vi "Trav_Prog_Extra_Commands.vi"() -> (1 "Extra Commands Array":string[](array[string]), 2 "Argument Examples":string[](array[string]))   [LabVIEW 2012]
uses:
  Globals/Extra_Commands_Global.vi
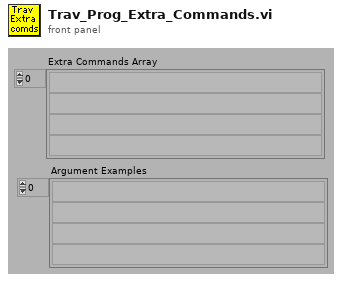
[diagram p1: front panel]
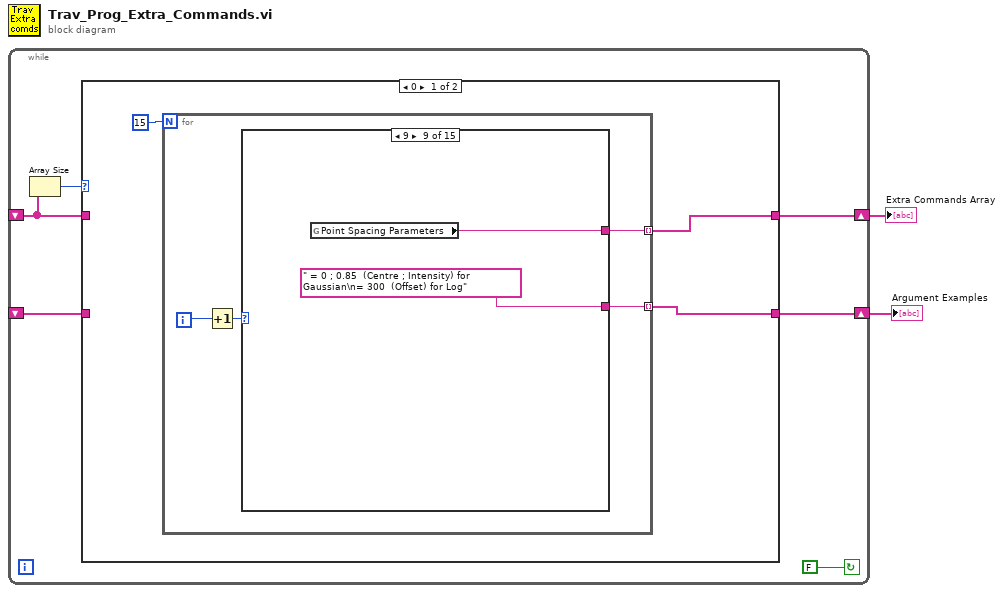
[diagram p0: block diagram]
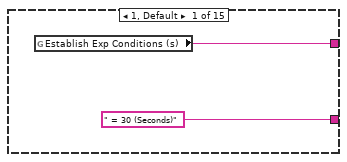
[diagram p2: hidden frame]
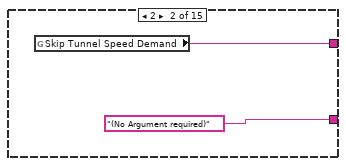
[diagram p3: hidden frame]
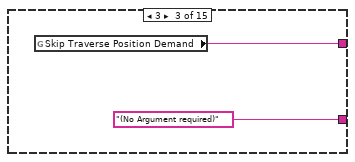
[diagram p4: hidden frame]
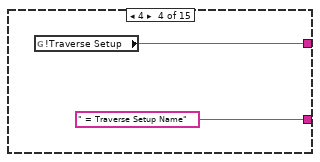
[diagram p5: hidden frame]
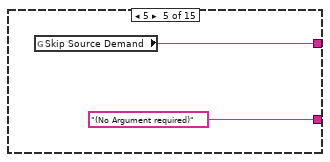
[diagram p6: hidden frame]
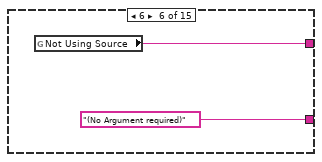
[diagram p7: hidden frame]
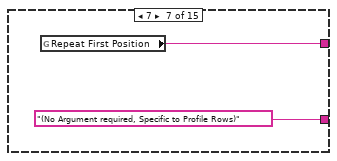
[diagram p8: hidden frame]
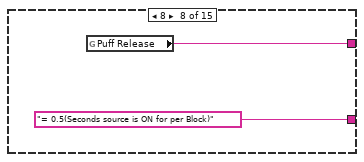
[diagram p9: hidden frame]
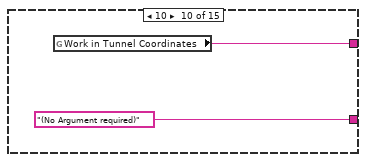
[diagram p10: hidden frame]
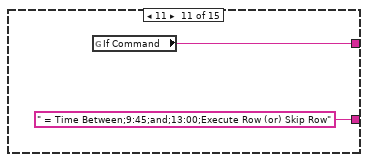
[diagram p11: hidden frame]
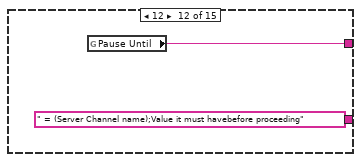
[diagram p12: hidden frame]
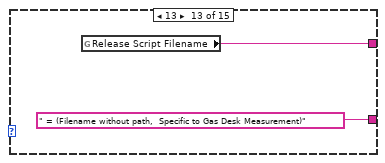
[diagram p13: hidden frame]
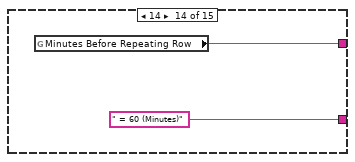
[diagram p14: hidden frame]
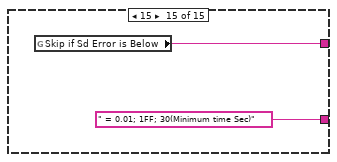
[diagram p15: hidden frame]
diagram:
  n1 = while {
    shift-left: _ -> [w4]
    shift-right: [w7] -> w1
    shift-left: _ -> [w5]
    shift-right: [w8] -> w2
    stop <- FALSE continue-if-true
    n2 = Array Size(array=w5) -> (size(s)=w6:i32)
    n3 = case shown="0" w6 {
      tunnel: [w10 w47] -> w8
      tunnel: [w9 w46] -> w7
      tunnel: w5 -> [_ w47]
      tunnel: w4 -> [_ w46]
      frame 0 {
        n4 = for {
          N: 15 -> [_]
          tunnel: [w13] -> w10 mode=indexing
          tunnel: [w12] -> w9 mode=indexing
          i -> [w15]
          n5 = Increment(x=w15) -> (x+1=w14:i32)
          n6 = case shown="9" w14 {
            tunnel: [w17 w19 w21 w23 w25 w27 w29 w31 w33 w35 w37 w39 w41 w43 w45] -> w13
            tunnel: [" = 30 (Seconds)" "(No Argument required)" "(No Argument required)" " = Traverse Setup Name" "(No Argument required)" "(No Argument required)" "(No Argument required, Specific to Profile Rows)" "= 0.5(Seconds source is ON for per Block)" " = 0 ; 0.85  (Centre ; Intensity) for Gaussian\n= 300  (Offset) for Log" "(No Argument required)" " = Time Between;9:45;and;13:00;Execute Row (or) Skip Row" " = (Server Channel name);Value it must havebefore proceeding" " = (Filename without path,  Specific to Gas Desk Measurement)" " = 60 (Minutes)" " = 0.01; 1FF; 30(Minimum time Sec)"] -> w12
            frame 1, Default {
              n7 = global read "Extra_Commands_Global.vi" "Establish Exp Conditions (s)"() -> (w17:string)
            }
            frame 2 {
              n8 = global read "Extra_Commands_Global.vi" "Skip Tunnel Speed Demand"() -> (w19:string)
            }
            frame 3 {
              n9 = global read "Extra_Commands_Global.vi" "Skip Traverse Position Demand"() -> (w21:string)
            }
            frame 4 {
              n10 = global read "Extra_Commands_Global.vi" "!Traverse Setup"() -> (w23:string)
            }
            frame 5 {
              n11 = global read "Extra_Commands_Global.vi" "Skip Source Demand"() -> (w25:string)
            }
            frame 6 {
              n12 = global read "Extra_Commands_Global.vi" "Not Using Source"() -> (w27:string)
            }
            frame 7 {
              n13 = global read "Extra_Commands_Global.vi" "Repeat First Position"() -> (w29:string)
            }
            frame 8 {
              n14 = global read "Extra_Commands_Global.vi" "Puff Release"() -> (w31:string)
            }
            frame 9 {
              n15 = global read "Extra_Commands_Global.vi" "Point Spacing Parameters"() -> (w33:string)
            }
            frame 10 {
              n16 = global read "Extra_Commands_Global.vi" "Work in Tunnel Coordinates"() -> (w35:string)
            }
            frame 11 {
              n17 = global read "Extra_Commands_Global.vi" "If Command"() -> (w37:string)
            }
            frame 12 {
              n18 = global read "Extra_Commands_Global.vi" "Pause Until"() -> (w39:string)
            }
            frame 13 {
              n19 = global read "Extra_Commands_Global.vi" "Release Script Filename"() -> (w41:string)
            }
            frame 14 {
              n20 = global read "Extra_Commands_Global.vi" "Minutes Before Repeating Row"() -> (w43:string)
            }
            frame 15 {
              n21 = global read "Extra_Commands_Global.vi" "Skip if Sd Error is Below"() -> (w45:string)
            }
          }
        }
      }
      frame 1, Default {
      }
    }
  }
  "Extra Commands Array" <- w2
  "Argument Examples" <- w1
